vi "ORS_CursorToCropIdx.vi"(8 "index offset":i32, 11 "Cursor List":T1=[{"Name"="img start", "Color"=16776960, "Style"=8, "Point Style"=13, "Name Visible"=FALSE, "Allow Drag"=TRUE, "Cursor Mode"=0, "Plot"=0, "Index"=0, "Position"={"X"=0.0, "Y"=50000.0}, "X Scale"=0, "Y Scale"=0, "Watch Plots"=[], "Watch All Plots"=FALSE, "Plot Area"=0, "Label Offset"={"X"=0.0, "Y"=5693.779904306226}}, {"Name"="img stop", "Color"=16776960, "Style"=8, "Point Style"=13, "Name Visible"=FALSE, "Allow Drag"=TRUE, "Cursor Mode"=0, "Plot"=0, "Index"=0, "Position"={"X"=4095.0, "Y"=50000.0}, "X Scale"=0, "Y Scale"=0, "Watch Plots"=[], "Watch All Plots"=FALSE, "Plot Area"=0, "Label Offset"={"X"=-1.7615894039736304, "Y"=6076.5550239234435}}, {"Name"="recal start", "Color"=16711680, "Style"=8, "Point Style"=13, "Name Visible"=FALSE, "Allow Drag"=TRUE, "Cursor Mode"=0, "Plot"=0, "Index"=0, "Position"={"X"=0.0, "Y"=50000.0}, "X Scale"=0, "Y Scale"=0, "Watch Plots"=[], "Watch All Plots"=FALSE, "Plot Area"=0, "Label Offset"={"X"=0.0, "Y"=6076.5550239234435}}, {"Name"="recal stop", "Color"=16711680, "Style"=8, "Point Style"=13, "Name Visible"=FALSE, "Allow Drag"=TRUE, "Cursor Mode"=0, "Plot"=0, "Index"=0, "Position"={"X"=4095.0, "Y"=50000.0}, "X Scale"=0, "Y Scale"=0, "Watch Plots"=[], "Watch All Plots"=FALSE, "Plot Area"=0, "Label Offset"={"X"=-1.7615894039736304, "Y"=6459.330143540676}}]) -> (0 "length":i32=4095, 1 "offset":i32)   [LabVIEW 2024]
uses:
  <vilib>/Utility/miscctls.llb/LVCursorListTypeDef.ctl
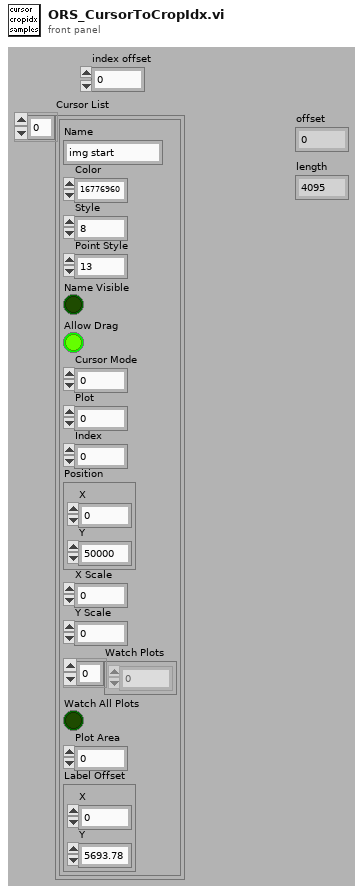
[diagram p1: front panel]
types:
  T1 = typedef "LVCursorListTypeDef.ctl" = cluster{"Name":string, "Color":u32, "Style":u8, "Point Style":u8, "Name Visible":bool, "Allow Drag":bool, "Cursor Mode":u32, "Plot":i32, "Index":i32, "Position":cluster{"X":dbl, "Y":dbl}, "X Scale":u32, "Y Scale":u32, "Watch Plots":i32[], "Watch All Plots":bool, "Plot Area":i32, "Label Offset":cluster{"X":dbl, "Y":dbl}}[]
  T2 = cluster{"Name":string, "Color":u32, "Style":u8, "Point Style":u8, "Name Visible":bool, "Allow Drag":bool, "Cursor Mode":u32, "Plot":i32, "Index":i32, "Position":cluster{"X":dbl, "Y":dbl}, "X Scale":u32, "Y Scale":u32, "Watch Plots":i32[], "Watch All Plots":bool, "Plot Area":i32, "Label Offset":cluster{"X":dbl, "Y":dbl}}
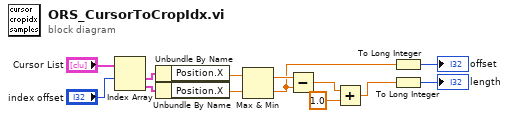
[diagram p0: block diagram]
diagram:
  n1 = Index Array(array="Cursor List", index #1="index offset") -> (element #1=w13:T2, element #2=w12:T2)  [unwired: 1 in]
  n2 = Unbundle By Name(w13) -> ("Position.X"=w11:dbl)
  n3 = Unbundle By Name(w12) -> ("Position.X"=w10:dbl)
  n4 = Max & Min(x=w11, y=w10) -> (max(x,y)=w9:dbl, min(x,y)=w6:dbl)
  n5 = Subtract(x=w9, y=w6) -> (x-y=w2:dbl)
  n6 = Add(x=w2, y=1.0) -> (x+y=w1:dbl)
  n7 = To Long Integer(number=w6) -> (32bit integer=→"offset":i32)
  n8 = To Long Integer(number=w1) -> (32bit integer=→"length":i32)
